vi "ErrorCodeDecoder(2).vi"(1 "array":string[][](array[string]), 2 "FTS Error Code In":i32) -> (0 "Error Message":string)   [LabVIEW 2013]
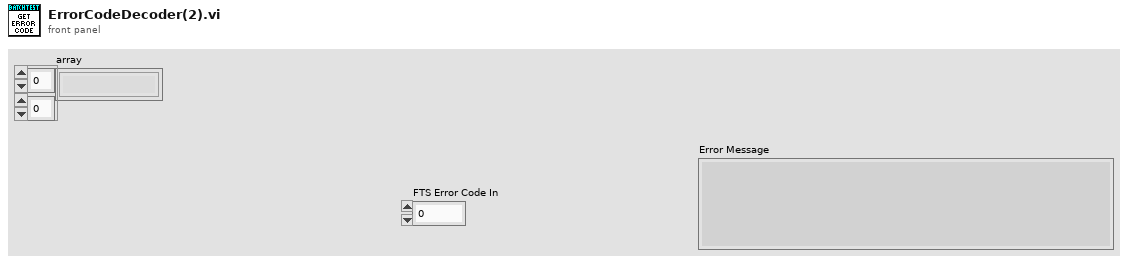
[diagram p1: front panel]
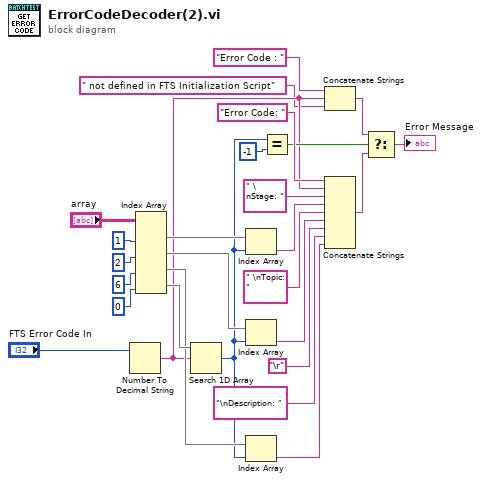
[diagram p0: block diagram]
diagram:
  n1 = Number To Decimal String(number="FTS Error Code In") -> (decimal integer string=w4:string)  [unwired: 1 in]
  n2 = Index Array(array="array", index (col) #1=1 ("disabled index (col)"), index (col) #2=2 ("index (col)"), index (col) #3=6 ("index (col)"), index (col) #4=0 ("index (col)")) -> (element #1=w18:string[], element #2=w19:string[], element #3=w20:string[], element #4=w21:string[])  [unwired: 4 in]
  n3 = Search 1D Array(1D array=w21, element=w4) -> (index of element=w9:i32)  [unwired: 1 in]
  n4 = Index Array(array=w18, index=w9) -> (element=w15:string)
  n5 = Index Array(array=w19, index=w9) -> (element=w13:string)
  n6 = Index Array(array=w20, index=w9) -> (element=w12:string)
  n7 = Equal?(x=w9, y=-1) -> (x = y?=w7:bool)
  n8 = Concatenate Strings("Error Code : " ("t"), w4, " not defined in FTS Initialization Script" ("string")) -> (w2:string)
  n9 = Concatenate Strings("Error Code: " ("string"), w4, " \nStage: " ("string"), w15, " \nTopic: " ("string"), w13, "\r", "\nDescription: " ("string"), w12) -> (w6:string)
  n10 = Select(t=w2, s=w7, f=w6) -> (s? t:f=→"Error Message":string)
